vi "open.vi"(8 "error in (no error)":errorcluster, 11 "PI P123.01 & PiezoDrive TD250 & NI USB 7855R in":refnum<class "PI P123.01 & PiezoDrive TD250 & NI USB 7855R.lvclass">) -> (0 "error out":errorcluster, 3 "PI P123.01 & PiezoDrive TD250 & NI USB 7855R out":refnum<class "PI P123.01 & PiezoDrive TD250 & NI USB 7855R.lvclass">)   [LabVIEW 2020, in "PI P123.01 & PiezoDrive TD250 & NI USB 7855R.lvclass"]
uses:
  PI P123.01 & PiezoDrive TD250 & NI USB 7855R.lvclass
  <vilib>/FPGAPlugInAG/USB-7855R/niLvFpga_Open_USB-7855R.vi
  <vilib>/rvi/interface/common/dynamic/niFpgaDynamicAddResources.vi
  <vilib>/Utility/error.llb/Error Cluster From Error Code.vi
  <vilib>/rvi/errors/niLvFpgaAdjustHostInterfaceError.vi
  <vilib>/rvi/interface/nirviOpenFPGA/nirviOpenFPGA.xnode
  FPGA Bitfiles/afmcontrol_FPGATarget_FPGAmain_od6Q9YeVPLc.lvbitx
  FPGA main.vi
  <vilib>/rvi/interface/nirviReadWriteControl/nirviReadWriteControl.xnode
  NiFpgaLv.dll
  <vilib>/rvi/interface/Simulation/niFpgaSimulationCallBeginRW.vi
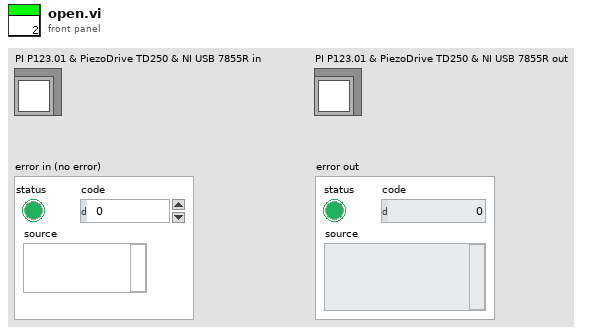
[diagram p1: front panel]
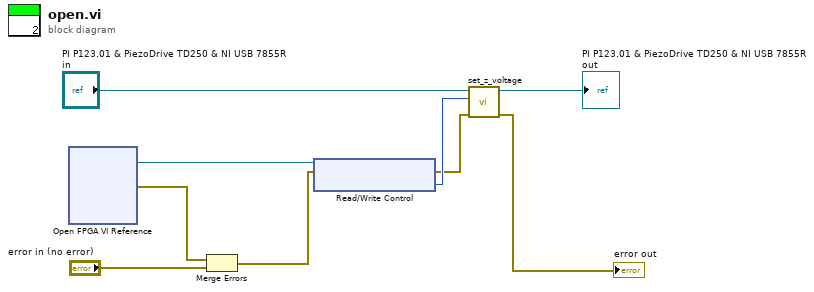
[diagram p0: block diagram]
diagram:
  n1 = xnode "Open FPGA VI Reference"() -> ("FPGA VI Reference Out"=w8:refnum<k20>, "error out"=w9:errorcluster)  [unwired: 2 in]
  n2 = Merge Errors(w9, "error in (no error)") -> (w7:errorcluster)
  n3 = xnode "Read/Write Control"("FPGA VI Reference In"=w8, "error in"=w7) -> ("error out"=w3:errorcluster, "PZT Z Control (Bits)"=w4:i16)  [unwired: 1 out]
  n4 = call-dynamic "set_z_voltage.vi"("error in (no error)"=w3, "Z voltage (bits)"=w4, "PI P123.01 & PiezoDrive TD250 & NI USB 7855R in"="PI P123.01 & PiezoDrive TD250 & NI USB 7855R in") -> ("error out"=→"error out":errorcluster, "PI P123.01 & PiezoDrive TD250 & NI USB 7855R out"=→"PI P123.01 & PiezoDrive TD250 & NI USB 7855R out":refnum<class "PI P123.01 & PiezoDrive TD250 & NI USB 7855R.lvclass">)  [unwired: 7 in]
